vi "Write TCP Logging.vi"(8 "error in (no error)":errorcluster, 10 "TCP Logging":bool, 11 "Dashboard Server in":refnum<class "Dashboard Server.lvclass">) -> (0 "error out":errorcluster, 3 "Dashboard Server out":refnum<class "Dashboard Server.lvclass">)   [LabVIEW 2019, in "Dashboard Server.lvclass"]
uses:
  Dashboard Server.lvclass
  Dashboard Server.lvclass/Dashboard Server.ctl
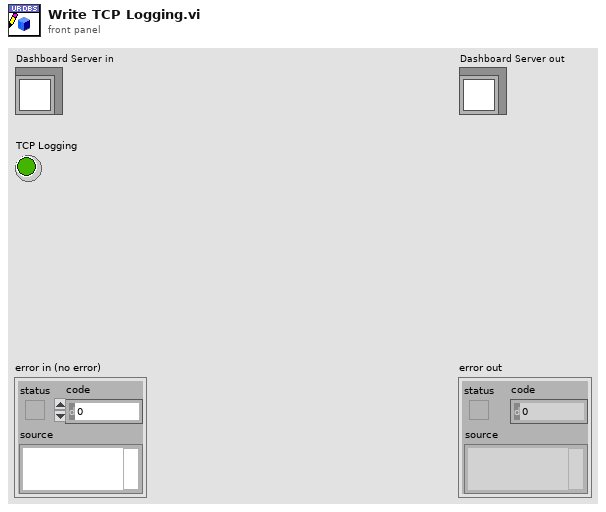
[diagram p1: front panel]
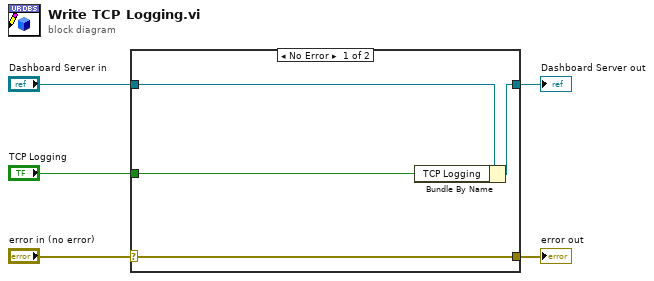
[diagram p0: block diagram]
diagram:
  n1 = case shown="No Error" "error in (no error)" {
    selector: "error in (no error)" -> [w9 w10]
    tunnel: [w9 w10] -> w4
    tunnel: [w7 w11] -> w2
    tunnel: "Dashboard Server in" -> [w8 w11]
    tunnel: "TCP Logging" -> [w6 _]
    frame No Error {
      n2 = Bundle By Name(cluster=w8, "TCP Logging"=w6) -> (w7:refnum<class "Dashboard Server.lvclass">)
    }
    frame Error {
    }
  }
  "error out" <- w4
  "Dashboard Server out" <- w2
